vi "bno055.vi"() -> ()   [LabVIEW 2019]
panel:
  out "x-y":dbl
  out "error out":errorcluster
  in  "error in (no error)":errorcluster
  out "dir":dbl
  in  "stop":bool
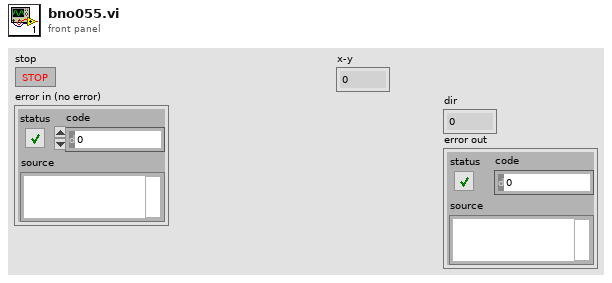
[diagram p1: front panel]
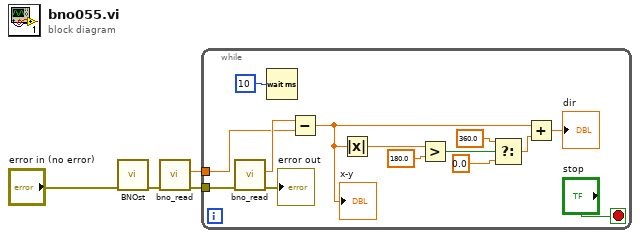
[diagram p0: block diagram]
diagram:
  n1 = call "BNOst.vi"("error in (no error)"="error in (no error)") -> ("error out"=w3:errorcluster)  [unwired: 10 in]
  n2 = call "bno_read.vi"("error in (no error)"=w3) -> ("error out"=w2:errorcluster, "x/y"=w1:dbl)  [unwired: 8 in]
  n3 = while {
    tunnel: w2 -> [w16]
    tunnel: w1 -> [w13]
    stop <- "stop" stop-if-true
    n4 = call "bno_read.vi"("error in (no error)"=w16) -> ("error out"=→"error out":errorcluster, "x/y"=w14:dbl)  [unwired: 8 in]
    n5 = Wait (ms)(milliseconds to wait=u32 10) -> ()  [unwired: 1 out]
    n6 = Subtract(x=w14, y=w13) -> (x-y=w7:dbl)
    "x-y" <- w7
    n7 = Absolute Value(x=w7) -> (abs(x)=w12:dbl)
    n8 = Greater?(x=w12, y=180.0) -> (0:w10:bool)
    n9 = Select(t=360.0, s=w10, f=0.0) -> (s? t:f=w6:dbl)
    n10 = Add(x=w7, y=w6) -> (x+y=→"dir":dbl)
  }
